vi "Test Case, Is One IPG Found.vi"() -> ()   [LabVIEW 2010]
uses:
  Charger/Charger_Status Control.ctl
  Drivers/Charger Test Set/Charger_Input Control.ctl
panel:
  in  "MICS ID array 3":u32[](array[numeric])=[1, 2, 57005] format="%.0x"
  in  "MICS ID array 2":u32[](array[numeric])=[48879] format="%.0x"
  in  "MICS ID array 1":u32[](array[numeric]) format="%.0x"
  in  "error in":errorcluster
  out "found one IPG3":bool
  out "found one IPG2":bool
  out "found one IPG1":bool
  in  "Charge Status 3":T1={"MICS ID"=4417, "VBAT"=nan, "ChargingState"="", "VBAT Slide"=3.5, "Status"="", "TemperatureLevel"=nan, "IPG_ReceivedLevel"=nan, "VBAT Target"=nan, "Charger Setpoint"=nan, "Index"=0, "Ready"=FALSE, "Charger Inputs"={"address"="COM17", "position"=0, "setpoint"=7500.0}, "MICS Inputs"={"address"="", "chan"=2, "ID"=0}} {"MICS Inputs"."ID" format="%04x"; "MICS Inputs"."chan" min=1 max=10 step=1; "Charger Inputs"."setpoint" min=0.0 max=20000.0 step=100.0; "Charger Inputs"."position" min=0 max=5 step=1; "MICS ID" format="%04x"; "VBAT Target" format="%.2f"; "VBAT Slide" scale=3.5..4.0 scale format="%.2f"; "VBAT" format="%.2f"}
  out "error out":errorcluster
  in  "Charge Status 2":T1={"MICS ID"=4417, "VBAT"=nan, "ChargingState"="", "VBAT Slide"=3.5, "Status"="", "TemperatureLevel"=nan, "IPG_ReceivedLevel"=nan, "VBAT Target"=nan, "Charger Setpoint"=nan, "Index"=0, "Ready"=FALSE, "Charger Inputs"={"address"="COM17", "position"=0, "setpoint"=7500.0}, "MICS Inputs"={"address"="", "chan"=2, "ID"=0}} {"MICS Inputs"."ID" format="%04x"; "MICS Inputs"."chan" min=1 max=10 step=1; "Charger Inputs"."setpoint" min=0.0 max=20000.0 step=100.0; "Charger Inputs"."position" min=0 max=5 step=1; "MICS ID" format="%04x"; "VBAT Target" format="%.2f"; "VBAT Slide" scale=3.5..4.0 scale format="%.2f"; "VBAT" format="%.2f"}
  in  "Charge Status 1":T1={"MICS ID"=4417, "VBAT"=nan, "ChargingState"="", "VBAT Slide"=3.5, "Status"="", "TemperatureLevel"=nan, "IPG_ReceivedLevel"=nan, "VBAT Target"=nan, "Charger Setpoint"=nan, "Index"=0, "Ready"=FALSE, "Charger Inputs"={"address"="COM17", "position"=0, "setpoint"=7500.0}, "MICS Inputs"={"address"="", "chan"=2, "ID"=0}} {"MICS Inputs"."ID" format="%04x"; "MICS Inputs"."chan" min=1 max=10 step=1; "Charger Inputs"."setpoint" min=0.0 max=20000.0 step=100.0; "Charger Inputs"."position" min=0 max=5 step=1; "MICS ID" format="%04x"; "VBAT Target" format="%.2f"; "VBAT Slide" scale=3.5..4.0 scale format="%.2f"; "VBAT" format="%.2f"}
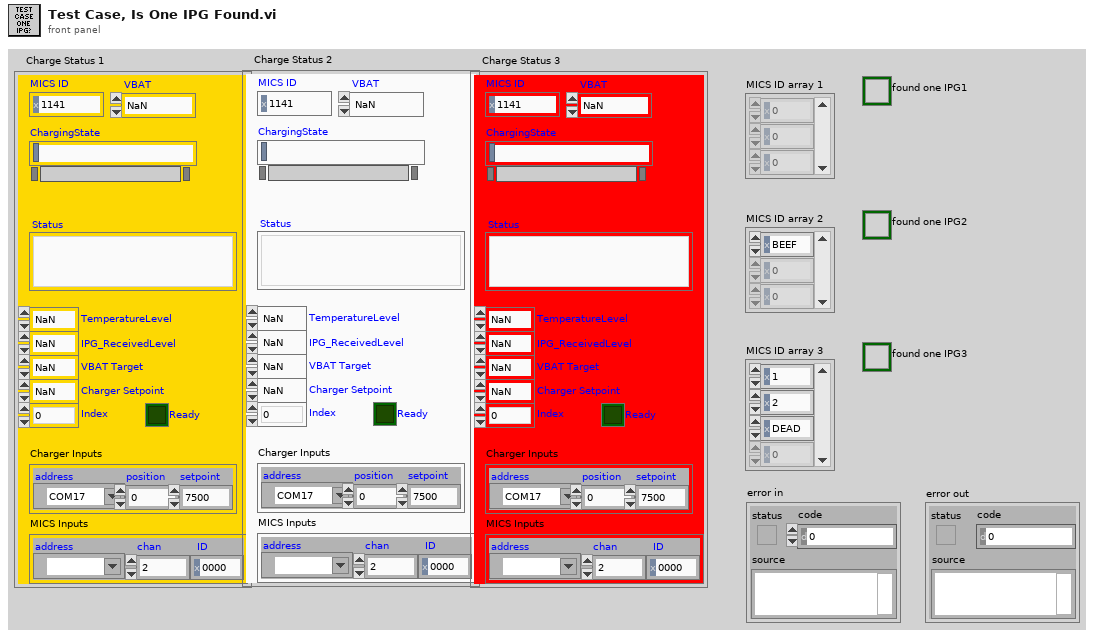
[diagram p1: front panel]
types:
  T1 = typedef "Charger_Status Control.ctl" = cluster{"MICS ID":u32, "VBAT":dbl, "ChargingState":string, "VBAT Slide":dbl, "Status":string, "TemperatureLevel":dbl, "IPG_ReceivedLevel":dbl, "VBAT Target":dbl, "Charger Setpoint":dbl, "Index":i32, "Ready":bool, "Charger Inputs":T2, "MICS Inputs":cluster{"address":refnum<visa-resource-name>, "chan":u16, "ID":u32}}
  T2 = typedef "Charger_Input Control.ctl" = cluster{"address":refnum<visa-resource-name>, "position":i32, "setpoint":dbl}
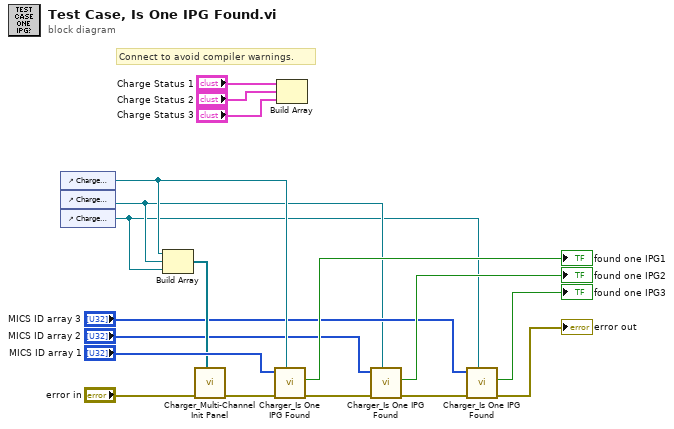
[diagram p0: block diagram]
diagram:
  # "Connect to avoid compiler warnings."
  n1 = control-ref of="Charge Status 1"() -> (w12:refnum<vi>)
  n2 = control-ref of="Charge Status 2"() -> (w2:refnum<vi>)
  n3 = control-ref of="Charge Status 3"() -> (w1:refnum<vi>)
  n4 = Build Array(w12, w2, w1) -> (w11:refnum<vi>[])
  n5 = call "Charger_Multi-Channel Init Panel.vi"("Status Refnum  Array"=w11, "error in"="error in") -> ("error out"=w9:errorcluster)  [unwired: 7 in]
  n6 = call "Charger_Is One IPG Found.vi"("Status Refnum"=w12, "error in"=w9, "MICS ID array"="MICS ID array 1") -> ("error out"=w8:errorcluster, "found one IPG"=→"found one IPG1":bool)  [unwired: 4 in, 1 out]
  n7 = Build Array("Charge Status 1", "Charge Status 2", "Charge Status 3") -> ()  [unwired: 1 out]
  n8 = call "Charger_Is One IPG Found.vi"("Status Refnum"=w2, "error in"=w8, "MICS ID array"="MICS ID array 2") -> ("error out"=w4:errorcluster, "found one IPG"=→"found one IPG2":bool)  [unwired: 4 in, 1 out]
  n9 = call "Charger_Is One IPG Found.vi"("Status Refnum"=w1, "error in"=w4, "MICS ID array"="MICS ID array 3") -> ("error out"=→"error out":errorcluster, "found one IPG"=→"found one IPG3":bool)  [unwired: 4 in, 1 out]
